vi "Deliver Request.vi"(8 "error in (no error)":errorcluster, 10 "Request":refnum<class "request.lvclass">, 11 "output_poller in":refnum<class "output_poller.lvclass">) -> (0 "error out":errorcluster, 3 "output_poller out":refnum<class "output_poller.lvclass">)   [LabVIEW 2015, in "output_poller.lvclass"]
uses:
  output_poller.lvclass
  Request/request.lvclass
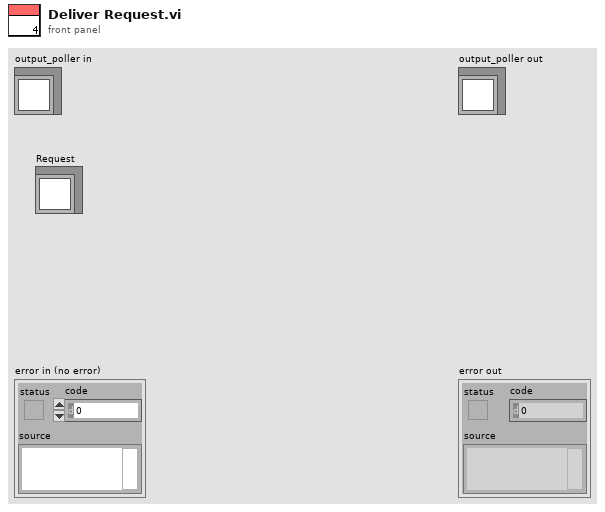
[diagram p1: front panel]
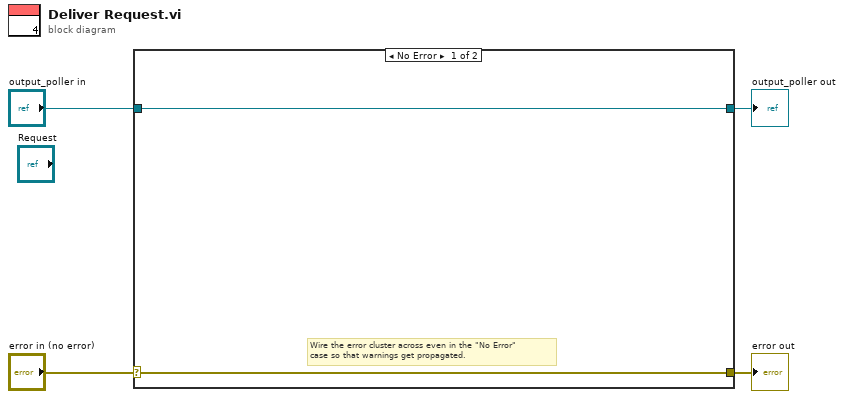
[diagram p0: block diagram]
diagram:
  n1 = case shown="No Error" "error in (no error)" {
    selector: "error in (no error)" -> [w5 w8]
    tunnel: [w5 w8] -> w3
    tunnel: [w6 w7] -> w1
    tunnel: "output_poller in" -> [w6 w7]
    frame No Error {
      # "Wire the error cluster across even in the \"No Error\"\ncase so that warnings get propagated."
    }
    frame Error {
    }
  }
  "error out" <- w3
  "output_poller out" <- w1
